vi "Measures of Mean.vi"(6 "percent (trim)":dbl=25.0, 10 "type":T1(ring), 11 "x array":dbl[](array[numeric])) -> (0 "error":i32, 3 "mean value":dbl)   [LabVIEW 2014, in "NI_Gmath.lvlib"]
doc: "Computes the central tendency of the data values in <B>x array</B>."
uses:
  NI_Gmath.lvlib
  Mean (DBL).vi
  NI_AALBase.lvlib
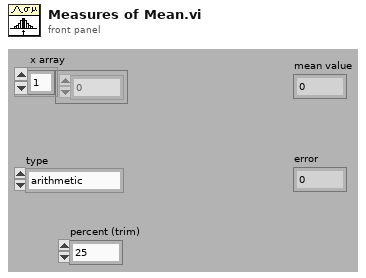
[diagram p1: front panel]
types:
  T1 = enum16{"arithmetic", "geometric", "harmonic", "trimmed", "median"}
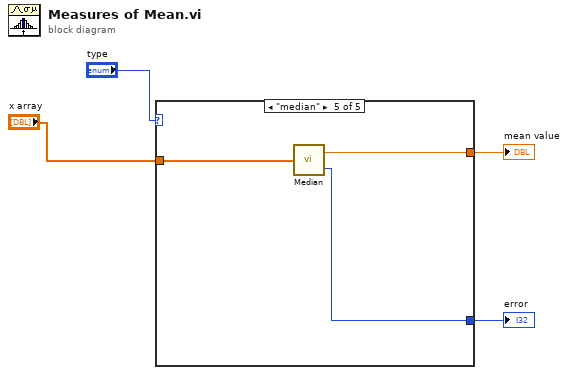
[diagram p0: block diagram]
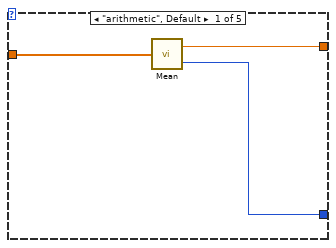
[diagram p2: hidden frame]
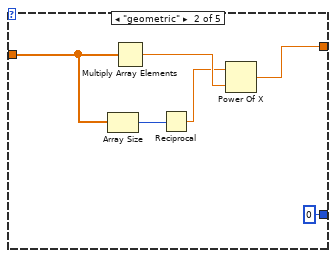
[diagram p3: hidden frame]
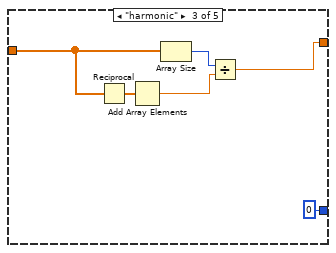
[diagram p4: hidden frame]
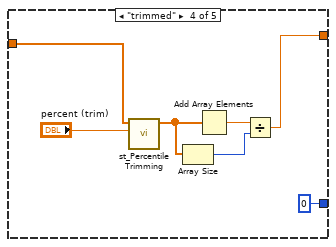
[diagram p5: hidden frame]
diagram:
  n1 = case shown="\"median\"" "type" {
    tunnel: "x array" -> [w7 w13 w19 w26 w29]
    tunnel: [w6 w9 w15 w20 w28] -> w2
    tunnel: [w5 0 ("error") 0 ("error") 0 ("error") w27] -> w1
    frame "arithmetic", Default {
      n2 = call-poly "Mean.vi"("X"=w7) -> ("mean"=w6:dbl, "error"=w5:i32)
    }
    frame "geometric" {
      n3 = Array Size(array=w13) -> (size(s)=w12:i32)
      n4 = Multiply Array Elements(1:w13) -> (0:w11:dbl)
      n5 = Reciprocal(x=w12) -> (1/x=w10:dbl)
      n6 = Power Of X(1:w11, 2:w10) -> (0:w9:dbl)
    }
    frame "harmonic" {
      n7 = Reciprocal(x=w19) -> (1/x=w18:dbl[])
      n8 = Add Array Elements(numeric array=w18) -> (sum=w16:dbl)
      n9 = Array Size(array=w19) -> (size(s)=w17:i32)
      n10 = Divide(x=w17, y=w16) -> (x/y=w15:dbl)
    }
    frame "trimmed" {
      n11 = call "st_Percentile Trimming.vi"("p"="percent (trim)", "x array"=w26) -> ("trimmed x array"=w24:dbl[])  [unwired: 9 in]
      n12 = Array Size(array=w24) -> (size(s)=w22:i32)
      n13 = Add Array Elements(numeric array=w24) -> (sum=w23:dbl)
      n14 = Divide(x=w23, y=w22) -> (x/y=w20:dbl)
    }
    frame "median" {
      n15 = call "Median.vi"("X"=w29) -> ("median"=w28:dbl, "error"=w27:i32)
    }
  }
  "mean value" <- w2
  "error" <- w1
